vi "Frequency Response Function (Mag-Phase) N-M.vi"(0 "time signals X":waveform(dbl)[](array[waveform]), 1 "restart averaging (F)":bool, 2 "window parameter":dbl=nan, 5 "time signals Y":waveform(dbl)[](array[waveform]), 7 "window":T1=1 items=["Rectangle"=0, "Hanning"=1, "Hamming"=2, "Blackman-Harris"=3, "Exact Blackman"=4, "Blackman"=5, "Flat Top"=6, "4 Term B-Harris "=7, "7 Term B-Harris"=8, "Low Sidelobe"=9, "Blackman Nuttall"=11, "Triangle"=30, "Bartlett-Hanning"=31, "Bohman"=32, "Parzen"=33, "Welch"=34, "Kaiser"=60, "Dolph-Chebyshev"=61, "Gaussian"=62], 9 "view":T3, 11 "error in (no error)":errorcluster, 12 "averaging parameters":T2={"averaging mode"=enum."No averaging", "weighting mode"=enum."Exponential", "number of averages"=10} {"number of averages" min=1}, 13 "FRF Mode":enum16{"H1", "H2", "H3"}(ring), 14 "X-Y pairing":enum32{"ordered pairs", "all cross pairs"}(ring)) -> (3 "averaging done":bool, 4 "magnitudes":cluster{"f0":dbl, "df":dbl, "magnitude":dbl[]}[](array[cluster]) {"magnitude" format="%.2p"; "f0" format="%0.2p"; "df" format="%0.2p"}, 6 "phases":cluster{"f0":dbl, "df":dbl, "phase":dbl[]}[](array[cluster]) {"phase" format="%.2p"; "f0" format="%0.2p"; "df" format="%0.2p"}, 8 "coherences":cluster{"f0":dbl, "df":dbl, "coherence":dbl[]}[](array[cluster]) {"coherence" format="%.2g"; "df" format="%.2g"; "f0" format="%.2g"}, 10 "averages completed":dbl format="%.2p", 15 "error out":errorcluster)   [LabVIEW 2020, in "NI_MAPro.lvlib"]
doc: "Computes the frequency response and the coherence based on the input signals. Results are returned as <B>magnitude</B>, <B>phase</B>, and <B>coherence</B>."
uses:
  NI_MAPro.lvlib
  windowTd.ctl
  2-chan State.ctl
  NI_MABase.lvlib
  NI_AALPro.lvlib
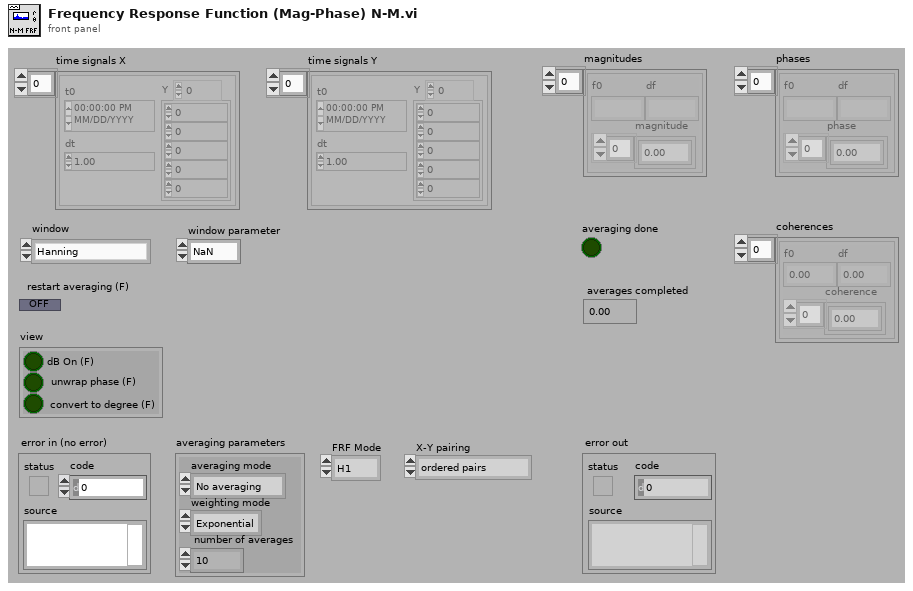
[diagram p1: front panel]
types:
  T1 = typedef "NI_AALPro.lvlib/windowTd.ctl" = u32
  T2 = cluster{"averaging mode":enum16{"No averaging", "Vector averaging", "RMS averaging", "Peak hold"}, "weighting mode":enum16{"Linear", "Exponential"}, "number of averages":u32}
  T3 = cluster{"dB On (F)":bool, "unwrap phase (F)":bool, "convert to degree (F)":bool}
  T4 = typedef "NI_MAPro.lvlib/2-chan State.ctl" = cluster{"Sx":cdb[], "Sy":cdb[], "Sxx":dbl[], "Syy":dbl[], "Sxy":cdb[], "block size":i32, "df":dbl, "dt":dbl, "avgs completed":dbl, "spectrum parameters":cluster{"averaging parameters":cluster{"averaging mode":enum16{"No averaging", "Vector averaging", "RMS averaging", "Peak hold"}, "weighting mode":enum16{"Linear", "Exponential"}, "number of averages":u32}, "window":T1}, "lin avg done":bool, "t0 history":dbl, "dt history":dbl, "timestamp":dbl}
  T5 = cluster{"f0":dbl, "df":dbl, "imag or phase":dbl[]}
  T6 = cluster{"f0":dbl, "df":dbl, "real or mag":dbl[]}[]
  T7 = cluster{"f0":dbl, "df":dbl, "imag or phase":dbl[]}[]
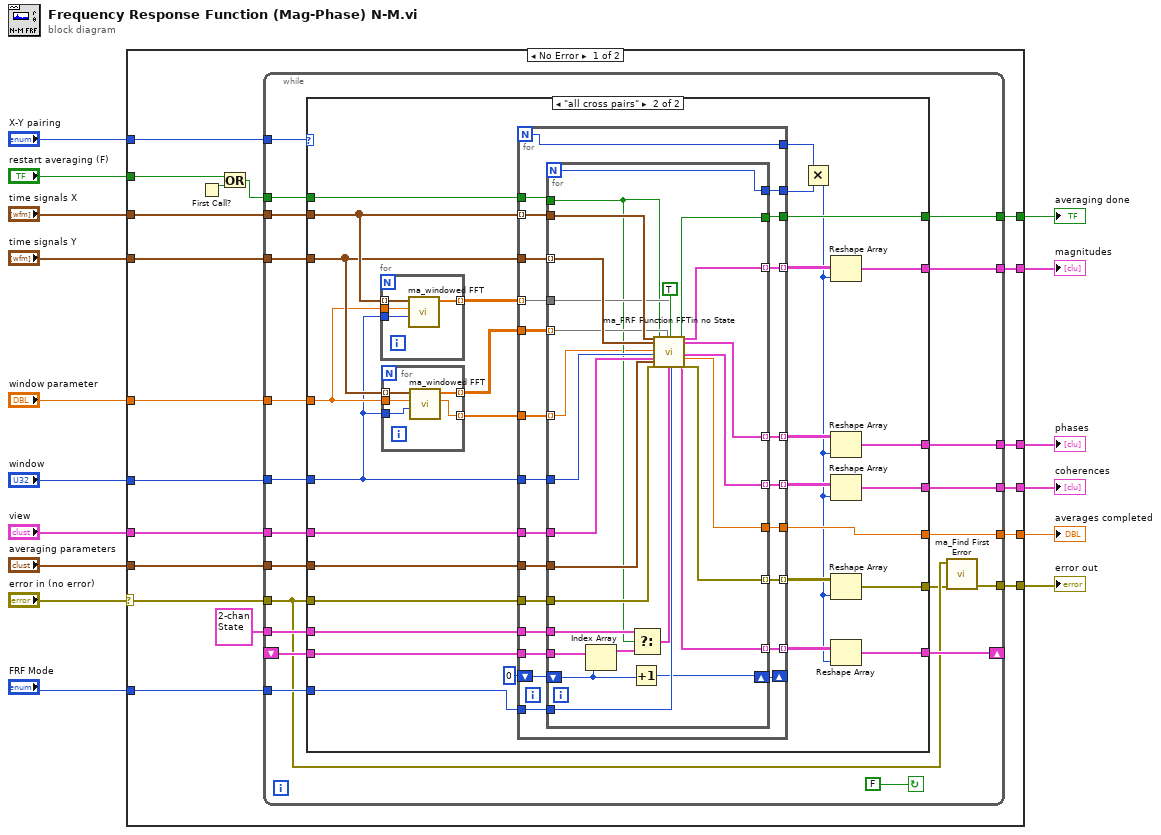
[diagram p0: block diagram]
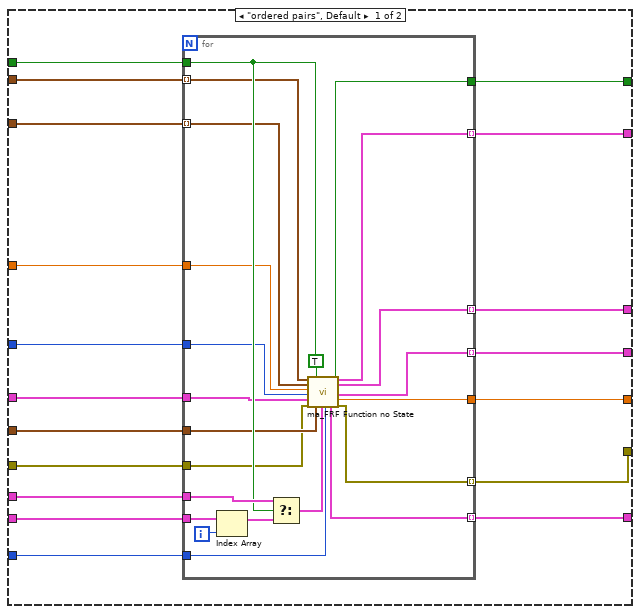
[diagram p2: hidden frame]
diagram:
  n1 = case shown="No Error" "error in (no error)" {
    selector: "error in (no error)" -> [w33 w186]
    tunnel: [w31 w186] -> w15
    tunnel: "FRF Mode" -> [w30 _]
    tunnel: "restart averaging (F)" -> [w29 _]
    tunnel: "time signals X" -> [w28 _]
    tunnel: "time signals Y" -> [w27 _]
    tunnel: "X-Y pairing" -> [w26 _]
    tunnel: "window" -> [w25 _]
    tunnel: "view" -> [w24 _]
    tunnel: "averaging parameters" -> [w23 _]
    tunnel: "window parameter" -> [w22 _]
    tunnel: [w21 _] -> w5
    tunnel: [w20 _] -> w4
    tunnel: [w19 _] -> w3
    tunnel: [w18 _] -> w2
    tunnel: [w17 _] -> w1
    frame No Error {
      n2 = First Call?() -> (First Call?: T/F=w35:bool)
      n3 = Or(x=w29, y=w35) -> (x .or. y?=w34:bool)
      n4 = while {
        tunnel: T4 {"Sx"=[], "Sy"=[], "Sxx"=[], "Syy"=[], "Sxy"=[], "block size"=0, "df"=0.0, "dt"=0.0, "avgs completed"=0.0, "spectrum parameters"={"averaging parameters"={"averaging mode"=enum."No averaging", "weighting mode"=enum."Linear", "number of averages"=0}, "window"=0}, "lin avg done"=FALSE, "t0 history"=0.0, "dt history"=0.0, "timestamp"=0.0} ("state info out") -> [w56]
        tunnel: w34 -> [w55]
        tunnel: w28 -> [w44]
        tunnel: w27 -> [w54]
        tunnel: w25 -> [w53]
        tunnel: w23 -> [w52]
        tunnel: w30 -> [w51]
        tunnel: [w50] -> w21
        tunnel: [w49] -> w17
        tunnel: w33 -> [w43]
        shift-right: [w47] -> _
        shift-left: _ -> [w46]
        tunnel: [w45] -> w31
        tunnel: [w42] -> w20
        tunnel: [w41] -> w19
        tunnel: [w40] -> w18
        tunnel: w26 -> [w38]
        tunnel: w24 -> [w37]
        tunnel: w22 -> [w36]
        stop <- FALSE continue-if-true
        n5 = case shown="\"all cross pairs\"" w38 {
          tunnel: w56 -> [w68 w126]
          tunnel: w55 -> [w74 w125]
          tunnel: w54 -> [w72 w102]
          tunnel: w53 -> [w71 w97]
          tunnel: w52 -> [w70 w124]
          tunnel: w51 -> [w66 w123]
          tunnel: [w59 w122] -> w50
          tunnel: [w63 w121] -> w49
          tunnel: [w65 w106] -> w47
          tunnel: w46 -> [w67 w120]
          tunnel: w44 -> [w73 w103]
          tunnel: w43 -> [w69 w119]
          tunnel: [w60 w115] -> w42
          tunnel: [w61 w112] -> w41
          tunnel: [w62 w111] -> w40
          tunnel: [w64 w109] -> w39
          tunnel: w37 -> [w58 w104]
          tunnel: w36 -> [w57 w101]
          frame "ordered pairs", Default {
            n6 = for {
              tunnel: w74 -> [w89]
              tunnel: [w96] -> w59
              tunnel: [w95] -> w63
              tunnel: [w94] -> w60 mode=indexing
              tunnel: [w91] -> w61 mode=indexing
              tunnel: w68 -> [w90]
              tunnel: w73 -> [w88] mode=indexing
              tunnel: w72 -> [w82] mode=indexing
              tunnel: w71 -> [w87]
              tunnel: w70 -> [w86]
              tunnel: w66 -> [w85]
              tunnel: [w84] -> w62 mode=indexing
              tunnel: w69 -> [w83]
              tunnel: [w81] -> w65 mode=indexing
              tunnel: w67 -> [w79]
              tunnel: [w77] -> w64 mode=indexing
              tunnel: w58 -> [w76]
              tunnel: w57 -> [w75]
              i -> [w80]
              n7 = Index Array(array=w79, index=w80) -> (element=w78:T4)
              n8 = Select(t=w90, s=w89, f=w78) -> (s? t:f=w93:T4)
              n9 = call "ma_FRF Function no State.vi"("time signal X"=w88, "time signal Y"=w82, "window parameter"=w75, "window"=w87, "view"=w76, "error in (no error)"=w83, "restart averaging (F)"=w89, "averaging parameters"=w86, "mag-phase"=TRUE, "state info"=w93, "FRF Mode"=w85) -> ("averaging done"=w96:bool, "state info out"=w81:T4, "real or mag"=w94:cluster{"f0":dbl, "df":dbl, "real or mag":dbl[]}, "imag or phase"=w91:T5, "coherence"=w84:cluster{"f0":dbl, "df":dbl, "coherence":dbl[]}, "averages completed"=w95:dbl, "error out"=w77:errorcluster)  [unwired: 2 out]
            }
          }
          frame "all cross pairs" {
            n10 = for {
              tunnel: w103 -> [w135] mode=indexing
              tunnel: [w134] -> w100 mode=indexing
              tunnel: w101 -> [w133]
              tunnel: w97 -> [w132]
              n11 = call "ma_windowed FFT.vi"("window"=w132, "window parameter"=w133, "time signal X"=w135) -> ("Sx"=w134:cdb[])  [unwired: 6 in, 2 out]
            }
            n12 = for {
              tunnel: w102 -> [w131] mode=indexing
              tunnel: [w130] -> w99 mode=indexing
              tunnel: w101 -> [w129]
              tunnel: [w128] -> w98 mode=indexing
              tunnel: w97 -> [w127]
              n13 = call "ma_windowed FFT.vi"("window"=w127, "window parameter"=w129, "time signal X"=w131) -> ("df"=w128:dbl, "Sx"=w130:cdb[])  [unwired: 6 in, 1 out]
            }
            n14 = for {
              N -> [w144]
              tunnel: w126 -> [w159]
              tunnel: w125 -> [w158]
              tunnel: w102 -> [w157]
              tunnel: w97 -> [w156]
              tunnel: w124 -> [w155]
              tunnel: w123 -> [w154]
              tunnel: [w153] -> w122
              tunnel: [w152] -> w121
              tunnel: [w151] -> w108 mode=indexing
              tunnel: w120 -> [w150]
              tunnel: w103 -> [w149] mode=indexing
              tunnel: w119 -> [w148]
              tunnel: [w147] -> w118 mode=indexing
              tunnel: [w146] -> w114 mode=indexing
              tunnel: [w145] -> w113 mode=indexing
              tunnel: [w144] -> w117
              tunnel: [w143] -> w116
              tunnel: [w142] -> w110 mode=indexing
              shift-right: [w140] -> _
              shift-left: 0 -> [w141]
              tunnel: w104 -> [w139]
              tunnel: w100 -> [w138] mode=indexing
              tunnel: w99 -> [w137]
              tunnel: w98 -> [w136]
              n15 = for {
                N -> [w169]
                tunnel: w158 -> [w162]
                tunnel: [w165] -> w153
                tunnel: [w185] -> w152
                tunnel: w159 -> [w182]
                tunnel: w149 -> [w181]
                tunnel: w157 -> [w177] mode=indexing
                tunnel: w156 -> [w173]
                tunnel: w155 -> [w180]
                tunnel: w154 -> [w179]
                tunnel: w148 -> [w178]
                tunnel: [w160] -> w151 mode=indexing
                tunnel: w150 -> [w176]
                tunnel: [w174] -> w142 mode=indexing
                tunnel: [w172] -> w147 mode=indexing
                tunnel: [w171] -> w146 mode=indexing
                tunnel: [w170] -> w145 mode=indexing
                tunnel: [w169] -> w143
                shift-right: [w167] -> w140
                shift-left: w141 -> [w168]
                tunnel: w139 -> [w166]
                tunnel: w138 -> [w164]
                tunnel: w137 -> [w163] mode=indexing
                tunnel: w136 -> [w161] mode=indexing
                n16 = Index Array(array=w176, index=w168) -> (element=w175:T4)
                n17 = Increment(x=w168) -> (x+1=w167:i32)
                n18 = Select(t=w182, s=w162, f=w175) -> (s? t:f=w184:T4)
                n19 = call "ma_FRF Function FFTin no State.vi"("time signal X"=w181, "time signal Y"=w177, "df"=w161, "window"=w173, "view"=w166, "error in (no error)"=w178, "restart averaging (F)"=w162, "averaging parameters"=w180, "mag-phase"=TRUE, "Sy"=w163, "state info"=w184, "Sx"=w164, "FRF Mode"=w179) -> ("averaging done"=w165:bool, "state info out"=w160:T4, "real or mag"=w172:cluster{"f0":dbl, "df":dbl, "real or mag":dbl[]}, "imag or phase"=w171:T5, "coherence"=w170:cluster{"f0":dbl, "df":dbl, "coherence":dbl[]}, "averages completed"=w185:dbl, "error out"=w174:errorcluster)  [unwired: 8 in]
              }
            }
            n20 = Multiply(x=w117, y=w116) -> (x*y=w107:i32)
            n21 = Reshape Array(w118, w107) -> (w115:T6)
            n22 = Reshape Array(w114, w107) -> (w112:T7)
            n23 = Reshape Array(w113, w107) -> (w111:cluster{"f0":dbl, "df":dbl, "coherence":dbl[]}[])
            n24 = Reshape Array(w110, w107) -> (w109:errorcluster[])
            n25 = Reshape Array(w108, w107) -> (w106:T4[])
          }
        }
        n26 = call "ma_Find First Error.vi"("error array in"=w39, "error in 1 (no error)"=w43) -> ("error out"=w45:errorcluster)  [unwired: 2 in, 3 out]
      }
    }
    frame Error {
    }
  }
  "error out" <- w15
  "averages completed" <- w1
  "averaging done" <- w5
  "coherences" <- w2
  "magnitudes" <- w4
  "phases" <- w3
